vi "Init YOLO.vi"(8 "error in (no error)":errorcluster, 9 "IoU":sgl=0.45, 10 "threshold":sgl=0.9, 11 "ONNX YOLO Class in":refnum<class "ONNX YOLO Class.lvclass">) -> (0 "error out":errorcluster, 3 "ONNX YOLO Class out":refnum<class "ONNX YOLO Class.lvclass">)   [LabVIEW 2017, in "ONNX YOLO Class Library.lvlib" / "ONNX YOLO Class.lvclass"]
uses:
  ONNX YOLO Class.lvclass
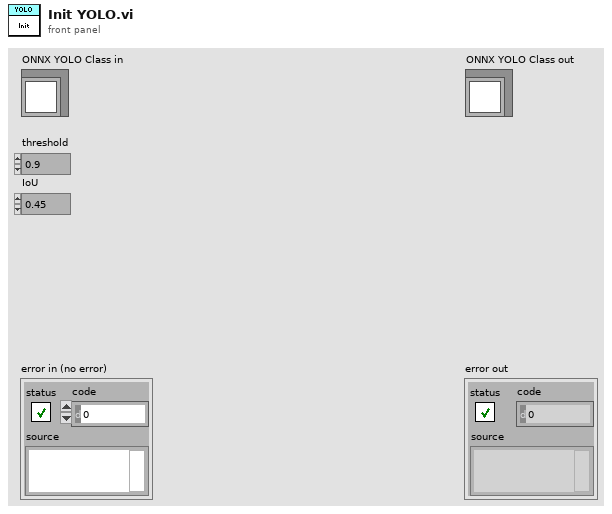
[diagram p1: front panel]
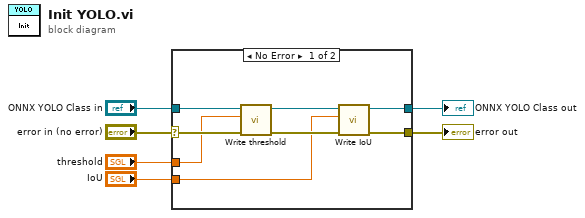
[diagram p0: block diagram]
diagram:
  n1 = case shown="No Error" "error in (no error)" {
    selector: "error in (no error)" -> [w11 w16]
    tunnel: [w9 w16] -> w5
    tunnel: [w12 w15] -> w3
    tunnel: "ONNX YOLO Class in" -> [w14 w15]
    tunnel: "threshold" -> [w8 _]
    tunnel: "IoU" -> [w7 _]
    frame No Error {
      n2 = call-dynamic "Write threshold.vi"("error in (no error)"=w11, "threshold"=w8, "ONNX YOLO Class in"=w14) -> ("error out"=w10:errorcluster, "ONNX YOLO Class out"=w13:refnum<class "ONNX YOLO Class.lvclass">)  [unwired: 7 in]
      n3 = call-dynamic "Write IoU.vi"("error in (no error)"=w10, "IoU"=w7, "ONNX YOLO Class in"=w13) -> ("error out"=w9:errorcluster, "ONNX YOLO Class out"=w12:refnum<class "ONNX YOLO Class.lvclass">)  [unwired: 7 in]
    }
    frame Error {
    }
  }
  "error out" <- w5
  "ONNX YOLO Class out" <- w3
